vi "_Spartan Version Tree.vi"   [LabVIEW 2011]
uses:
  SI.LIB/OGAB Version.ctl
  www/tests/PIM/LIB/PIM Version.vi
  www/tests/S Parameter/LIB/S Parameter Version.vi
  www/drivers/VNA/Rohde & Schwarz/LIB/Rohde & Schwarz VNA Version.vi
  www/drivers/VNA/Anritsu/LIB/Anritsu VNA Version.vi
  www/tests/Prompted Inputs/LIB/Prompted Inputs Version.vi
  www/client/client.lib/Spartan Client Version.vi
  www/drivers/VNA/Simulator/LIB/Simulator VNA Version.vi
  www/drivers/VNA/Agilent/LIB/Agilent VNA Version.vi
  www/drivers/SWI/Simulator/LIB/Simulator SWI Version.vi
  www/drivers/SWI/Sea-Level/LIB/Sea-Level SWI Version.vi
  www/tests/Prompt/LIB/Prompt Version.vi
  www/drivers/DMM/Agilent/LIB/Agilent DMM Version.vi
  server/server lib/Spartan Version.vi
  www/tests/DC Attenuation/LIB/DC Attenuation Version.vi
  www/drivers/DMM/Simulator/LIB/Simulator DMM Version.vi
panel:
  # "VERSION TREE"
types:
  T1 = typedef "OGAB Version.ctl" = cluster{"Version":string, "Build Number":u32, "Build Date/Time":dbl}
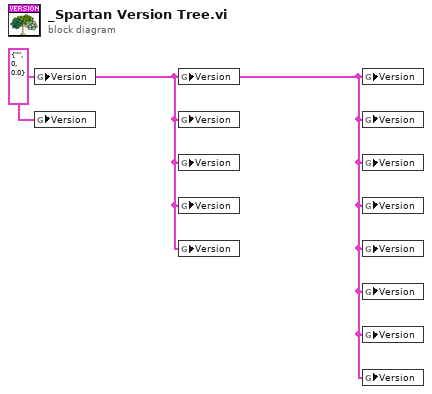
[diagram p0: block diagram]
diagram:
  w1 = T1 {"Version"="", "Build Number"=0, "Build Date/Time"=0.0} ("Version")
  n1 = global write "Spartan Version.vi" "Version"(w1) -> ()
  n2 = global write "Spartan Client Version.vi" "Version"(w1) -> ()
  n3 = global write "DC Attenuation Version.vi" "Version"(w1) -> ()
  n4 = global write "Prompt Version.vi" "Version"(w1) -> ()
  n5 = global write "S Parameter Version.vi" "Version"(w1) -> ()
  n6 = global write "Prompted Inputs Version.vi" "Version"(w1) -> ()
  n7 = global write "PIM Version.vi" "Version"(w1) -> ()
  n8 = global write "Agilent DMM Version.vi" "Version"(w1) -> ()
  n9 = global write "Simulator DMM Version.vi" "Version"(w1) -> ()
  n10 = global write "Sea-Level SWI Version.vi" "Version"(w1) -> ()
  n11 = global write "Simulator SWI Version.vi" "Version"(w1) -> ()
  n12 = global write "Agilent VNA Version.vi" "Version"(w1) -> ()
  n13 = global write "Simulator VNA Version.vi" "Version"(w1) -> ()
  n14 = global write "Anritsu VNA Version.vi" "Version"(w1) -> ()
  n15 = global write "Rohde & Schwarz VNA Version.vi" "Version"(w1) -> ()
